vi "Sensor Test.vi"(8 "error in (no error)":errorcluster, 11 "Test Type":string) -> (0 "Error Out":errorcluster, 2 "Error String":string, 3 "Passed?":bool)   [LabVIEW 2015]
uses:
  CAN Communication/Gas/Typedefs/Pressure Sensor.ctl
  CAN Communication/Gas/Gas.lvclass
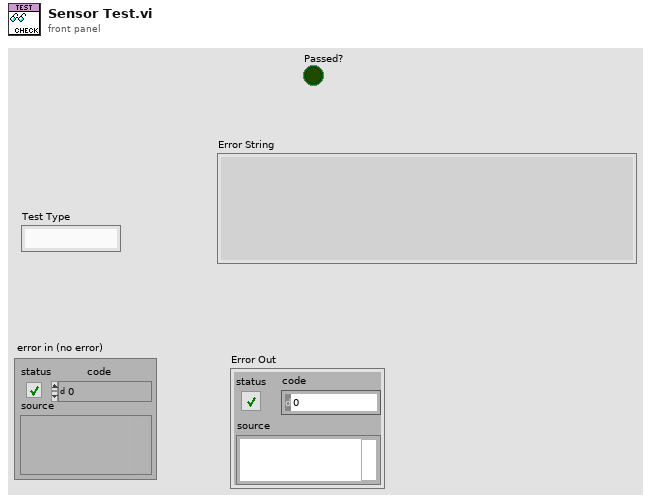
[diagram p1: front panel]
types:
  T1 = typedef "Gas.lvclass/Pressure Sensor.ctl" = u16
  T2 = typedef "Gas.lvclass/Session Handle.ctl" = refnum<data-value>
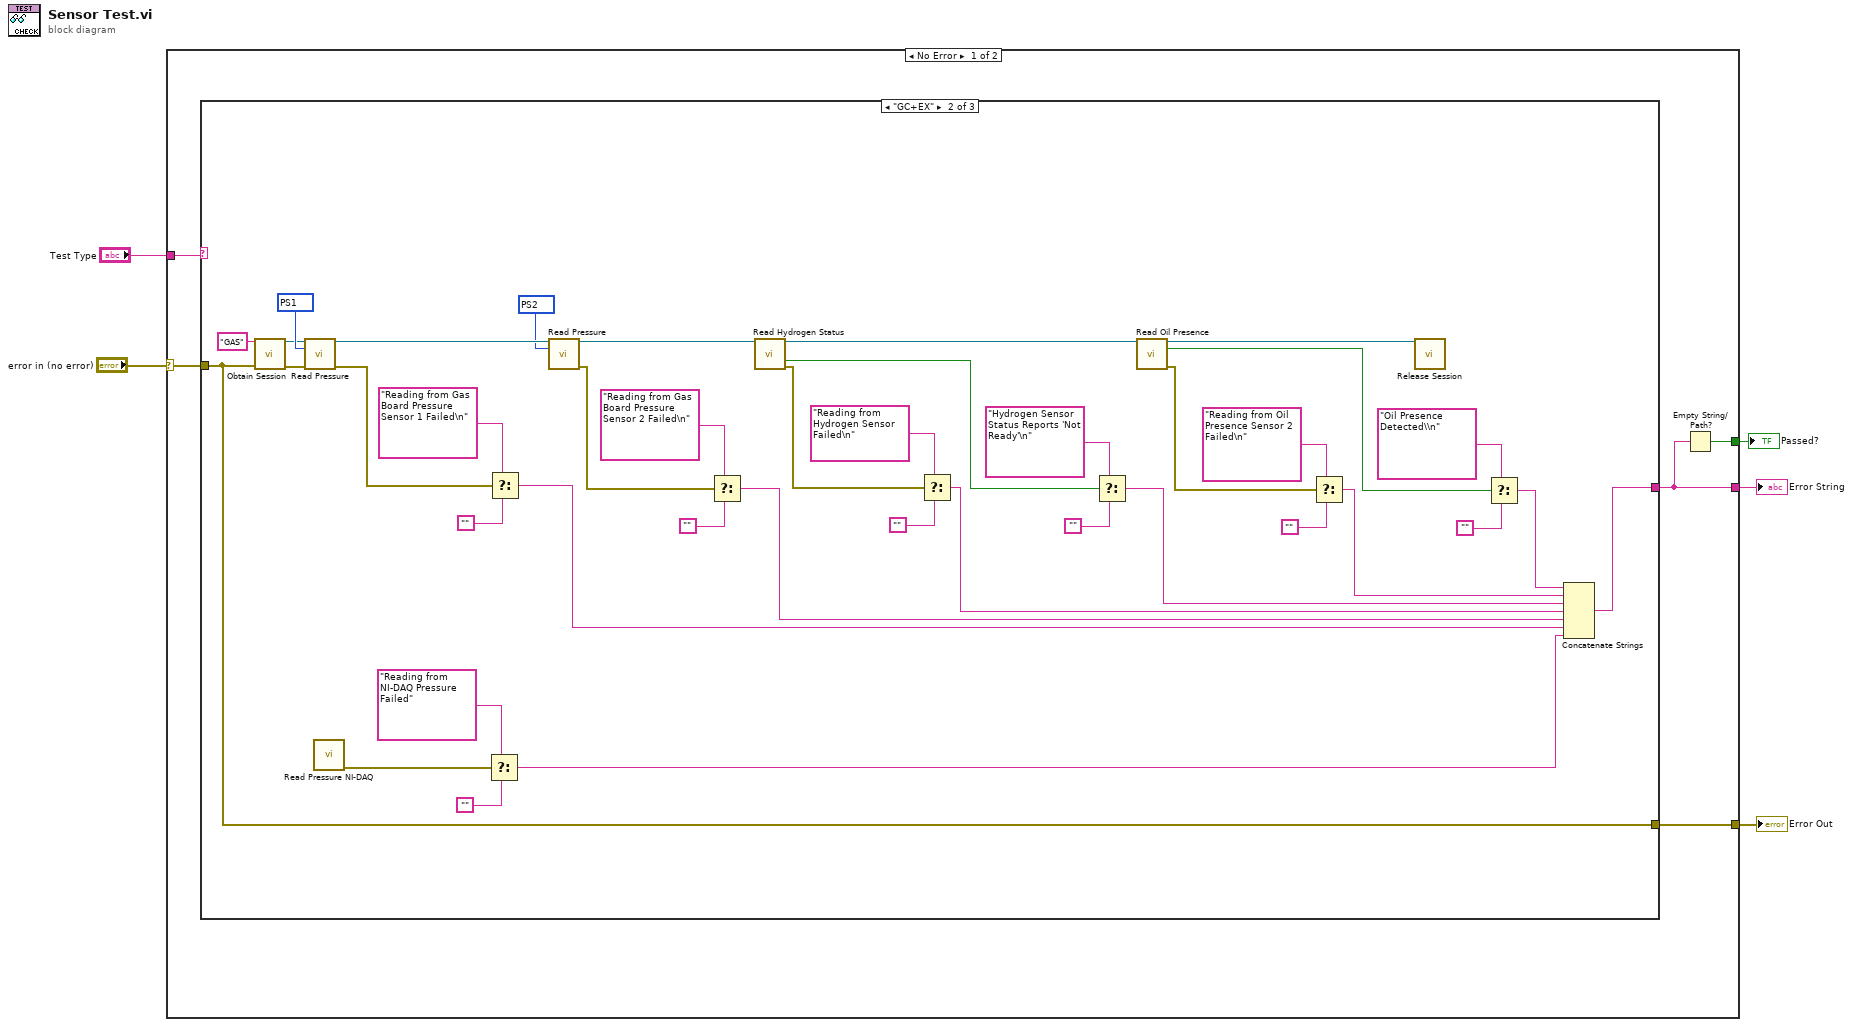
[diagram p0: block diagram]
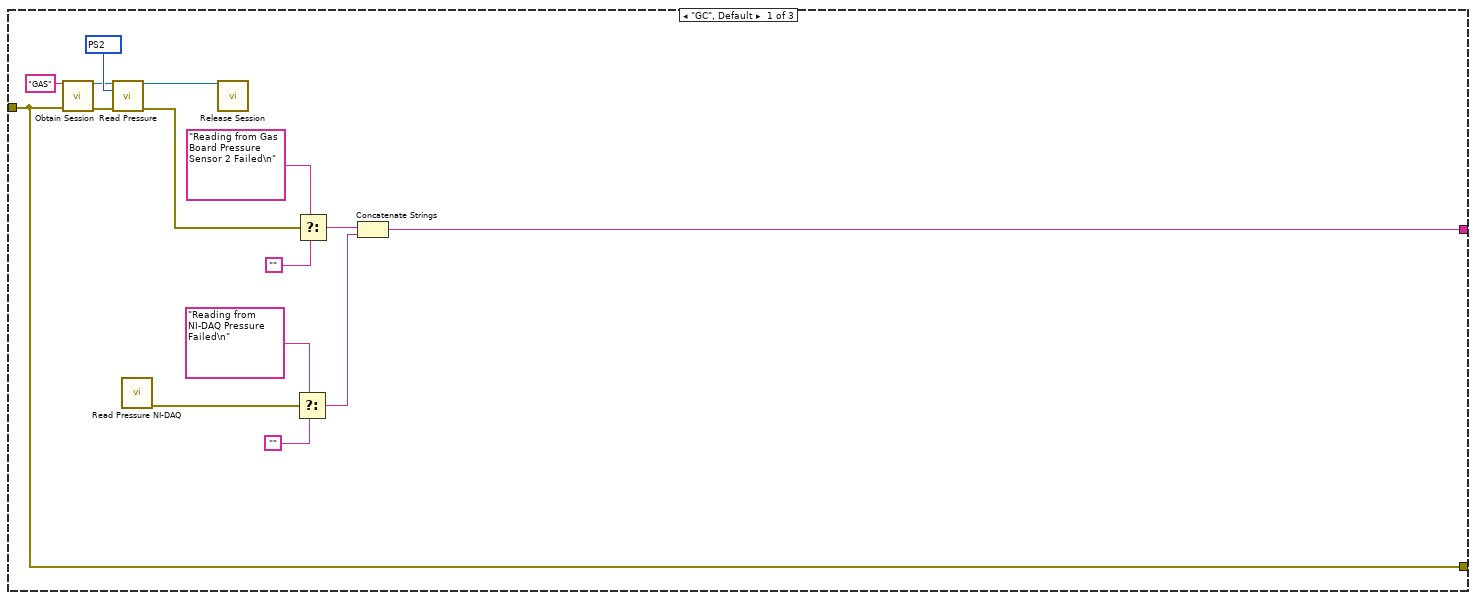
[diagram p2: hidden frame]
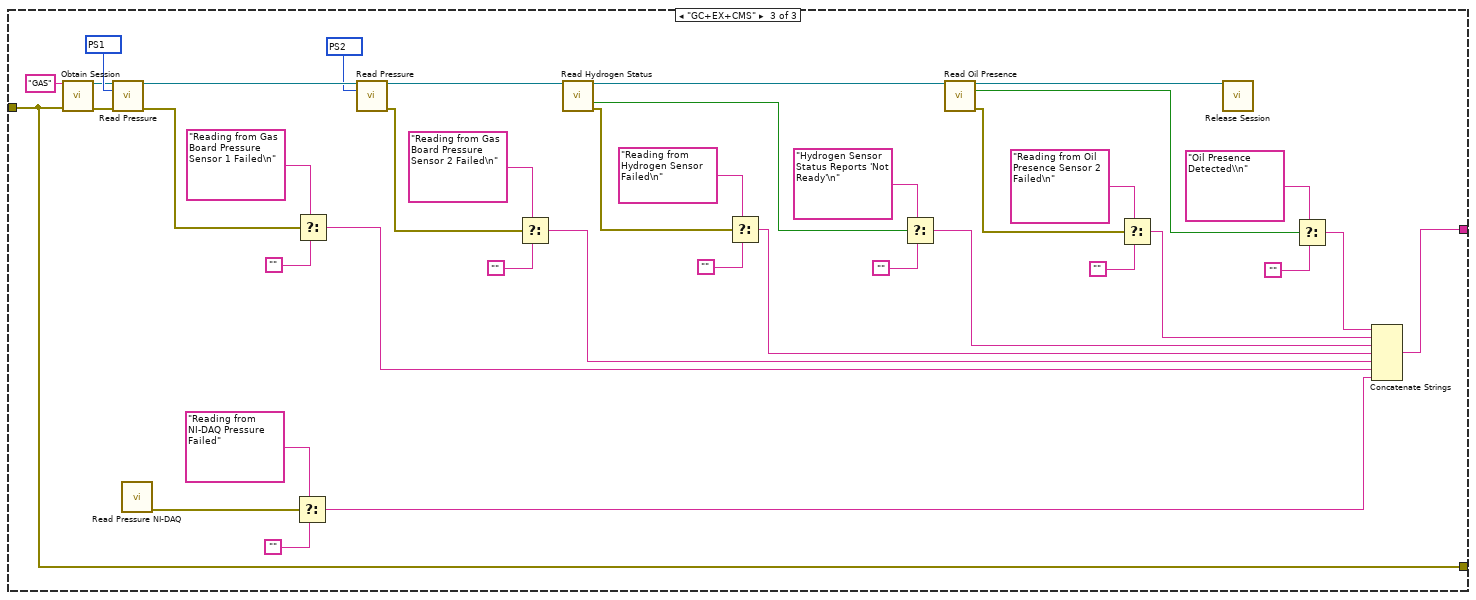
[diagram p3: hidden frame]
diagram:
  n1 = case shown="No Error" "error in (no error)" {
    selector: "error in (no error)" -> [w9 w104]
    tunnel: "Test Type" -> [w10 _]
    tunnel: [w7 _] -> w3
    tunnel: [w8 w104] -> w2
    tunnel: [w6 _] -> w1
    frame No Error {
      n2 = case shown="\"GC+EX\"" w10 {
        tunnel: w9 -> [w11 w26 w65]
        tunnel: [w12 w27 w66] -> w7
        tunnel: [w11 w26 w65] -> w8
        frame "GC", Default {
          w24 = T1 225 items=["PS1"=224, "PS2"=225] ("Pressure Sensor")
          n3 = call "Obtain Session.vi"("Session  Name ()"="GAS", "error in (no error)"=w11) -> ("Session Handle"=w23:T2, "error out"=w21:errorcluster)  [unwired: 12 in]
          n4 = call "Read Pressure.vi"("Session Handle in"=w23, "Pressure Sensor"=w24, "error in (no error)"=w21) -> ("Session Handle out"=w22:T2, "error out"=w20:errorcluster)  [unwired: 10 in, 1 out]
          n5 = call "Read Pressure NI-DAQ.vi"() -> ("error out"=w14:errorcluster)  [unwired: 10 in, 1 out]
          n6 = call "Release Session.vi"("Session Handle"=w22) -> ()  [unwired: 14 in, 1 out]
          n7 = Select(t="Reading from NI-DAQ Pressure Failed\n", s=w14, f="") -> (s? t:f=w13:string)
          n8 = Select(t="Reading from Gas Board Pressure Sensor 2 Failed\n", s=w20, f="") -> (s? t:f=w17:string)
          n9 = Concatenate Strings(w17, w13) -> (w12:string)
        }
        frame "GC+EX" {
          w51 = T1 225 items=["PS1"=224, "PS2"=225] ("Pressure Sensor")
          w63 = T1 224 items=["PS1"=224, "PS2"=225] ("Pressure Sensor")
          n10 = call "Obtain Session.vi"("Session  Name ()"="GAS", "error in (no error)"=w26) -> ("Session Handle"=w62:T2, "error out"=w61:errorcluster)  [unwired: 12 in]
          n11 = call "Read Pressure.vi"("Session Handle in"=w62, "Pressure Sensor"=w63, "error in (no error)"=w61) -> ("Session Handle out"=w52:T2, "error out"=w60:errorcluster)  [unwired: 10 in, 1 out]
          n12 = call "Read Pressure NI-DAQ.vi"() -> ("error out"=w55:errorcluster)  [unwired: 10 in, 1 out]
          n13 = Select(t="Reading from NI-DAQ Pressure Failed", s=w55, f="") -> (s? t:f=w28:string)
          n14 = Select(t="Reading from Gas Board Pressure Sensor 1 Failed\n", s=w60, f="") -> (s? t:f=w29:string)
          n15 = call "Read Pressure.vi"("Session Handle in"=w52, "Pressure Sensor"=w51) -> ("Session Handle out"=w49:T2, "error out"=w50:errorcluster)  [unwired: 11 in, 1 out]
          n16 = Select(t="Reading from Gas Board Pressure Sensor 2 Failed\n", s=w50, f="") -> (s? t:f=w30:string)
          n17 = call "Read Hydrogen Status.vi"("Session Handle in"=w49) -> ("Ready?"=w43:bool, "Session Handle out"=w42:T2, "error out"=w46:errorcluster)  [unwired: 9 in, 3 out]
          n18 = Select(t="Reading from Hydrogen Sensor Failed\n", s=w46, f="") -> (s? t:f=w31:string)
          n19 = Select(t="Hydrogen Sensor Status Reports 'Not Ready'\n", s=w43, f="") -> (s? t:f=w32:string)
          n20 = call "Read Oil Presence.vi"("Session Handle in"=w42) -> ("Session Handle out"=w35:T2, "Present?"=w36:bool, "error out"=w37:errorcluster)  [unwired: 12 in]
          n21 = Select(t="Reading from Oil Presence Sensor 2 Failed\n", s=w37, f="") -> (s? t:f=w33:string)
          n22 = call "Release Session.vi"("Session Handle"=w35) -> ()  [unwired: 14 in, 1 out]
          n23 = Select(t="Oil Presence Detected\\n", s=w36, f="") -> (s? t:f=w34:string)
          n24 = Concatenate Strings(w34, w33, w32, w31, w30, w29, w28) -> (w27:string)
        }
        frame "GC+EX+CMS" {
          w90 = T1 225 items=["PS1"=224, "PS2"=225] ("Pressure Sensor")
          w102 = T1 224 items=["PS1"=224, "PS2"=225] ("Pressure Sensor")
          n25 = call "Obtain Session.vi"("Session  Name ()"="GAS", "error in (no error)"=w65) -> ("Session Handle"=w101:T2, "error out"=w100:errorcluster)  [unwired: 12 in]
          n26 = call "Read Pressure.vi"("Session Handle in"=w101, "Pressure Sensor"=w102, "error in (no error)"=w100) -> ("Session Handle out"=w91:T2, "error out"=w99:errorcluster)  [unwired: 10 in, 1 out]
          n27 = call "Read Pressure NI-DAQ.vi"() -> ("error out"=w94:errorcluster)  [unwired: 10 in, 1 out]
          n28 = Select(t="Reading from NI-DAQ Pressure Failed", s=w94, f="") -> (s? t:f=w67:string)
          n29 = Select(t="Reading from Gas Board Pressure Sensor 1 Failed\n", s=w99, f="") -> (s? t:f=w68:string)
          n30 = call "Read Pressure.vi"("Session Handle in"=w91, "Pressure Sensor"=w90) -> ("Session Handle out"=w88:T2, "error out"=w89:errorcluster)  [unwired: 11 in, 1 out]
          n31 = Select(t="Reading from Gas Board Pressure Sensor 2 Failed\n", s=w89, f="") -> (s? t:f=w69:string)
          n32 = call "Read Hydrogen Status.vi"("Session Handle in"=w88) -> ("Ready?"=w82:bool, "Session Handle out"=w81:T2, "error out"=w85:errorcluster)  [unwired: 9 in, 3 out]
          n33 = Select(t="Reading from Hydrogen Sensor Failed\n", s=w85, f="") -> (s? t:f=w70:string)
          n34 = Select(t="Hydrogen Sensor Status Reports 'Not Ready'\n", s=w82, f="") -> (s? t:f=w71:string)
          n35 = call "Read Oil Presence.vi"("Session Handle in"=w81) -> ("Session Handle out"=w74:T2, "Present?"=w75:bool, "error out"=w76:errorcluster)  [unwired: 12 in]
          n36 = Select(t="Reading from Oil Presence Sensor 2 Failed\n", s=w76, f="") -> (s? t:f=w72:string)
          n37 = call "Release Session.vi"("Session Handle"=w74) -> ()  [unwired: 14 in, 1 out]
          n38 = Select(t="Oil Presence Detected\\n", s=w75, f="") -> (s? t:f=w73:string)
          n39 = Concatenate Strings(w73, w72, w71, w70, w69, w68, w67) -> (w66:string)
        }
      }
      n40 = Empty String/Path?(string/path=w7) -> (empty?=w6:bool)
    }
    frame Error {
    }
  }
  "Error String" <- w3
  "Error Out" <- w2
  "Passed?" <- w1
